vi "close_visa_resources.vi"(8 "error in (no error)":errorcluster, 11 "VISA in":T1) -> (0 "error out":errorcluster)   [LabVIEW 2015]
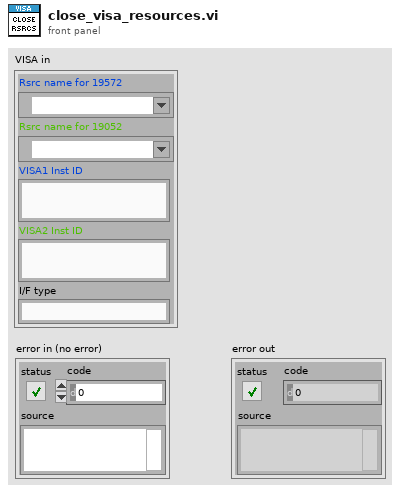
[diagram p1: front panel]
types:
  T1 = cluster{"Rsrc name for 19572":refnum<visa-resource-name>, "Rsrc name for 19052":refnum<visa-resource-name>, "I/F type":string, "VISA2 Inst ID":string, "VISA1 Inst ID":string}
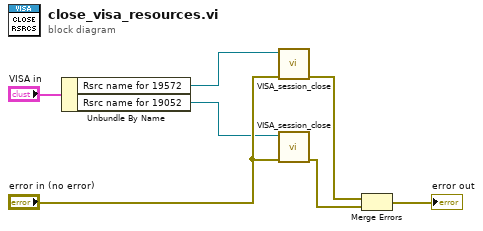
[diagram p0: block diagram]
diagram:
  n1 = Unbundle By Name("VISA in") -> ("Rsrc name for 19572"=w3:refnum<visa-resource-name>, "Rsrc name for 19052"=w2:refnum<visa-resource-name>)
  n2 = call "VISA_session_close.vi"("error in (no error)"="error in (no error)", "VISA resource name"=w3) -> ("error out"=w5:errorcluster)  [unwired: 8 in, 1 out]
  n3 = call "VISA_session_close.vi"("error in (no error)"="error in (no error)", "VISA resource name"=w2) -> ("error out"=w6:errorcluster)  [unwired: 8 in, 1 out]
  n4 = Merge Errors(w5, w6) -> (→"error out":errorcluster)
